vi "Winches Controller.vi"(8 "error in":errorcluster) -> ()   [LabVIEW 2019]
doc: "This VI executes continuously carrying out the current operation and responding to updates or new operations. It will often contain the timing or control code that is difficult to place directly in TeleOp. This VI generally opens all sensors and motors and isolates the rest of the robot code from knowing how the operations are carried out."
uses:
  <vilib>/Rock Robotics/WPI/Framework/Completion Status.ctl
  Winches Setpoints.ctl
  Winches Operations.ctl
  <vilib>/Rock Robotics/WPI/ThirdParty/Phoenix-LabVIEW/Motor Controller/Controls/CTRE_Phoenix_MotorControl_ControlMode.ctl
  Framework/Robot Global Data.vi
  <vilib>/Rock Robotics/Network Tables/NT Write Boolean.vi
panel:
  in  "Interactive Values":T1={"Operation"=enum."Actuate Lift", "Percent Power"=0.0}
  out "Current\nCmd":string
  in  "Buttons":cluster{"Execute Cmd":bool, "Abort Cmd":bool}
  out "Command Timing":cluster{"Start Time (ms)":u32, "Iterations":i32}
  out "Status":T3
  # "Tip: It may be helpful to observe inputs and sensor values.\nYou may also want to display tuning or debugging controls."
  # "Interactive Command: You may fill in the settings for a command\nand schedule it with the Execute button. You can observe and abort\nany command while fine tuning the code for the controller."
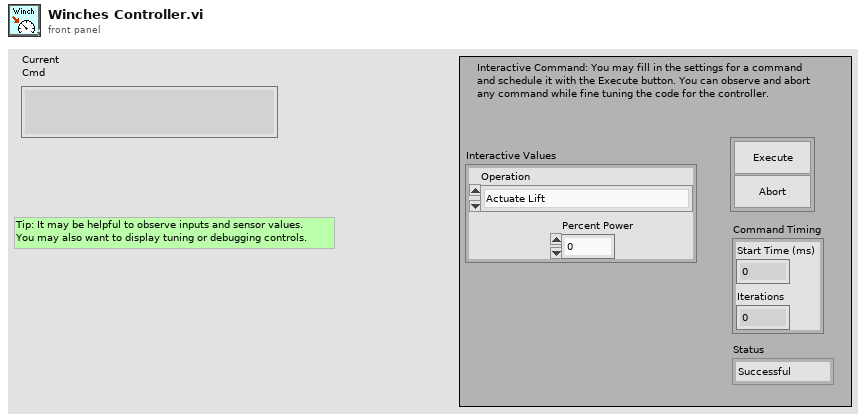
[diagram p1: front panel]
types:
  T1 = typedef "Winches Setpoints.ctl" = cluster{"Operation":T2, "Percent Power":dbl}
  T2 = typedef "Winches Operations.ctl" = enum16{"Reserve", "Read Current", "Actuate Lift", "Actuate Telescope"}
  T3 = typedef "Completion Status.ctl" = enum16{"Successful", "Aborted", "Incomplete"}
  T4 = typedef "WPI_MotorControlDeviceRef.ctl" = cluster{"DeviceStatus":errorcluster, "Type":T5, "PWM":cluster{"PWM Channel":T6, "DeadBand":T7}, "CAN":cluster{"Device Number":u8, "SetOutput VI Ref":variant, "GetOutput VI Ref":variant, "Enable VI Ref":variant, "Disable VI Ref":variant, "Data":variant}, "Invert":bool, "DIO PWM":cluster{"PWM \"Enable\" Channel":T6, "DIOChannel":T8, "PWM Rate":dbl}}
  T5 = typedef "WPI_MotorControlType.ctl" = enum16{"PWM", "CAN", "DIO PWM"}
  T6 = typedef "FPGA_DIOPWMChannel.ctl" = enum8{"PWM 0", "PWM 1", "PWM 2", "PWM 3", "PWM 4", "PWM 5", "PWM 6", "PWM 7", "PWM 8", "PWM 9", "PWM MXP 0", "PWM MXP 1", "PWM MXP 2", "PWM MXP 3", "PWM MXP 4", "PWM MXP 5", "PWM MXP 6", "PWM MXP 7", "PWM MXP 8", "PWM MXP 9", "Invalid"}
  T7 = typedef "WPI_PWMDeadband.ctl" = cluster{"Name":string, "maxPositivePwm":i32, "minPositivePwm":i32, "centerPwm":i32, "maxNegativePwm":i32, "minNegativePwm":i32, "angularRange":u16}
  T8 = typedef "FPGA_DIOChannel.ctl" = enum8{"DIO 0", "DIO 1", "DIO 2", "DIO 3", "DIO 4", "DIO 5", "DIO 6", "DIO 7", "DIO 8", "DIO 9", "DIO MXP 0", "DIO MXP 1", "DIO MXP 2", "DIO MXP 3", "DIO MXP 4", "DIO MXP 5", "DIO MXP 6", "DIO MXP 7", "DIO MXP 8", "DIO MXP 9", "DIO MXP 10", "DIO MXP 11", "DIO MXP 12", "DIO MXP 13", "DIO MXP 14", "DIO MXP 15", "SPI Port CS1", "SPI Port CS2", "SPI Port CS3", "SPI Port MISO", "SPI Port MOSI", "Invalid"}
  T9 = typedef "Command Status Info.ctl" = cluster{"Name":string, "Status":T3, "notifier out":T10}
  T10 = typedef "Completion Notifier.ctl" = refnum<notifier>
  T11 = cluster{"Current Command":T1, "Command Timing":cluster{"Start Time (ms)":u32, "Iterations":i32}, "Command Arguments":cluster{"Command Info":T9, "Description":string, "Default Command":T1, "queue out":refnum<queue>, "Subsystem Name":string}}
  T12 = typedef "CTRE_Phoenix_MotorControl_ControlMode.ctl" = u16
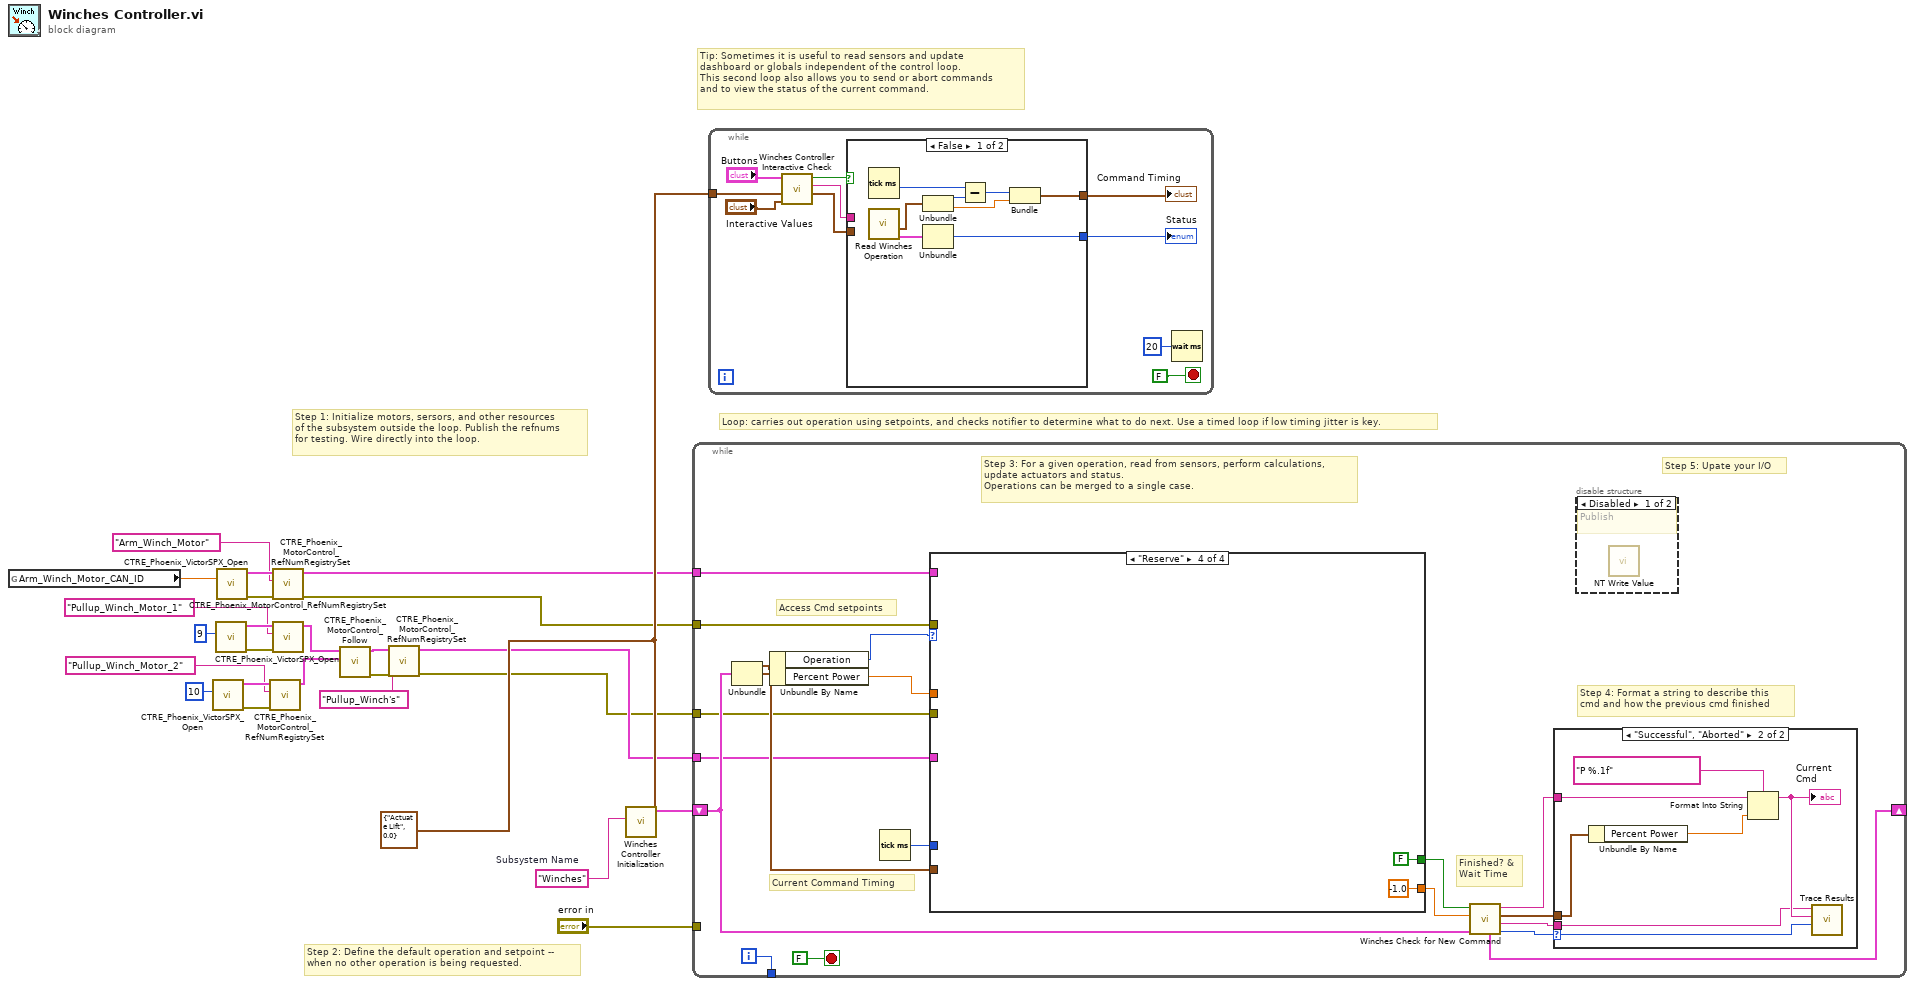
[diagram p0: block diagram]
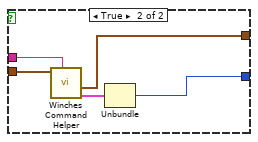
[diagram p2: hidden frame]
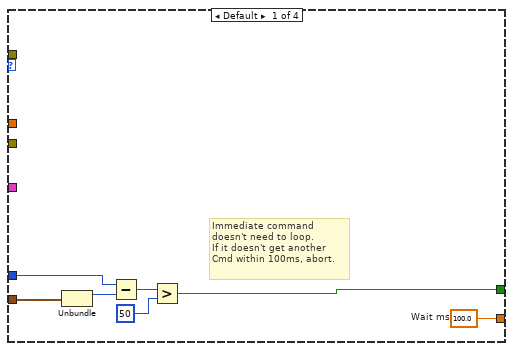
[diagram p5: hidden frame]
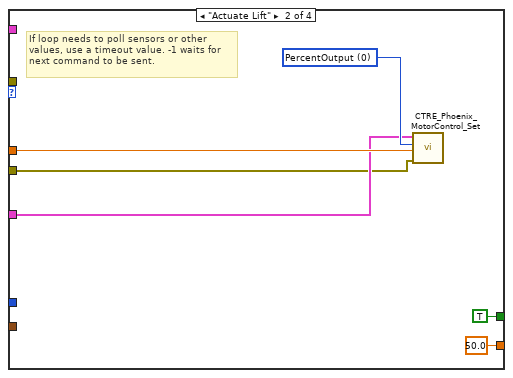
[diagram p6: hidden frame]
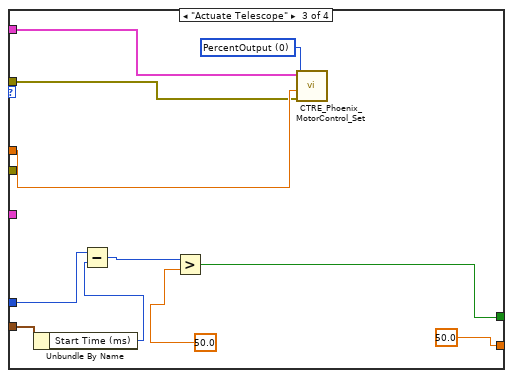
[diagram p7: hidden frame]
diagram:
  w12 = T1 {"Operation"=enum."Actuate Lift", "Percent Power"=0.0} ("Default Command")
  w23 = "Winches"  # Subsystem Name
  # "Tip: Sometimes it is useful to read sensors and update\ndashboard or globals independent of the control loop.\nThis second loop also allows you to send or abort commands\nand to view the status of the current command."
  # "Step 2: Define the default operation and setpoint --\nwhen no other operation is being requested."
  # "Step 1: Initialize motors, sersors, and other resources\nof the subsystem outside the loop. Publish the refnums\nfor testing. Wire directly into the loop."
  # "Loop: carries out operation using setpoints, and checks notifier to determine what to do next. Use a timed loop if low timing jitter is key."
  n1 = global read "Robot Global Data.vi" "Arm_Winch_Motor_CAN_ID"() -> (w22:dbl)
  n2 = call <vilib>:"CTRE_Phoenix_VictorSPX_Open.vi"("Device Number"=u8 10) -> ("error out"=w17:errorcluster, "CAN Talon SRX Ref"=w16:T4)  [unwired: 9 in]
  n3 = call <vilib>:"CTRE_Phoenix_VictorSPX_Open.vi"("Device Number"=u8 9) -> ("error out"=w19:errorcluster, "CAN Talon SRX Ref"=w18:T4)  [unwired: 9 in]
  n4 = call <vilib>:"CTRE_Phoenix_VictorSPX_Open.vi"("Device Number"=w22) -> ("error out"=w21:errorcluster, "CAN Talon SRX Ref"=w20:T4)  [unwired: 9 in]
  n5 = call <vilib>:"CTRE_Phoenix_MotorControl_RefNumRegistrySet.vi"("error in (no error)"=w17, "refnum name"="Pullup_Winch_Motor_2", "PhoenixMotorControlDevRef"=w16) -> ("PhoenixMotorControlDevRef"=w6:T4)  [unwired: 7 in, 1 out]
  n6 = call <vilib>:"CTRE_Phoenix_MotorControl_RefNumRegistrySet.vi"("error in (no error)"=w21, "refnum name"="Arm_Winch_Motor", "PhoenixMotorControlDevRef"=w20) -> ("error out"=w10:errorcluster, "PhoenixMotorControlDevRef"=w11:T4)  [unwired: 7 in]
  n7 = call <vilib>:"CTRE_Phoenix_MotorControl_RefNumRegistrySet.vi"("error in (no error)"=w19, "refnum name"="Pullup_Winch_Motor_1", "PhoenixMotorControlDevRef"=w18) -> ("PhoenixMotorControlDevRef"=w7:T4)  [unwired: 7 in, 1 out]
  n8 = call <vilib>:"CTRE_Phoenix_MotorControl_Follow.vi"("Master Controller to Follow"=w6, "PhoenixMotorControlDevRef"=w7) -> ("error out"=w5:errorcluster, "PhoenixMotorControlDevRef"=w4:T4)  [unwired: 8 in]
  n9 = call <vilib>:"CTRE_Phoenix_MotorControl_RefNumRegistrySet.vi"("error in (no error)"=w5, "refnum name"="Pullup_Winch's", "PhoenixMotorControlDevRef"=w4) -> ("error out"=w2:errorcluster, "PhoenixMotorControlDevRef"=w3:T4)  [unwired: 7 in]
  n10 = call "Winches Controller Initialization.vi"("Subsystem Name"=w23, "Default Command"=w12) -> ("Current Command"=w24:T11)  [unwired: 9 in]
  n11 = while {
    shift-right: [w40] -> _
    shift-left: w24 -> [w33]
    tunnel: [w43] -> _
    tunnel: "error in" -> [_]
    tunnel: w11 -> [w30]
    tunnel: w10 -> [w29]
    tunnel: w3 -> [w27]
    tunnel: w2 -> [w26]
    i -> [w43]
    stop <- FALSE stop-if-true
    # "Step 5: Upate your I/O"
    # "Step 4: Format a string to describe this\ncmd and how the previous cmd finished"
    # "Current Command Timing"
    # "Access Cmd setpoints"
    # "Finished? &\nWait Time"
    # "Step 3: For a given operation, read from sensors, perform calculations,\nupdate actuators and status.\nOperations can be merged to a single case."
    n12 = Unbundle(w33) -> ("Current Command"=w32:T1, "Command Timing"=w41:cluster{"Start Time (ms)":u32, "Iterations":i32})  [unwired: 1 out]
    n13 = Unbundle By Name(w32) -> ("Operation"=w31:T2, "Percent Power"=w28:dbl)
    n14 = Tick Count (ms)() -> (millisecond timer value=w42:u32)
    n15 = case shown="\"Reserve\"" w31 {
      tunnel: [w58 50.0 ("Wait ms") 50.0 -1.0 ("Wait ms")] -> w38
      tunnel: [w52 TRUE w71 FALSE] -> w39
      tunnel: w41 -> [w54 _ w69 _]
      tunnel: w42 -> [w53 _ w73 _]
      tunnel: w28 -> [_ w63 w75 _]
      tunnel: w30 -> [_ _ w66 _]
      tunnel: w29 -> [_ _ w65 _]
      tunnel: w27 -> [_ w60 _ _]
      tunnel: w26 -> [_ w59 _ _]
      frame Default {
        w58 = 100.0  # Wait ms
        # "Immediate command\ndoesn't need to loop.\nIf it doesn't get another\nCmd within 100ms, abort."
        n16 = Unbundle(w54) -> ("Start Time (ms)"=w57:u32)  [unwired: 1 out]
        n17 = Subtract(x=w53, y=w57) -> (x-y=w56:u32)
        n18 = Greater?(x=w56, y=u8 50 ("Left Motor")) -> (0:w52:bool)
      }
      frame "Actuate Lift" {
        w64 = T12 0 items=["PercentOutput"=0, "Position"=1, "Velocity"=2, "Current"=3, "Follower"=5, "MotionProfile"=6, "MotionMagic"=7, "MotionProfileArc"=10, "Disabled"=15] ("Control Mode")
        # "If loop needs to poll sensors or other\nvalues, use a timeout value. -1 waits for\nnext command to be sent."
        n19 = call <vilib>:"CTRE_Phoenix_MotorControl_Set.vi"("error in (no error)"=w59, "Output"=w63, "Control Mode"=w64, "PhoenixMotorControlDevRef"=w60) -> ()  [unwired: 6 in, 2 out]
      }
      frame "Actuate Telescope" {
        w74 = T12 0 items=["PercentOutput"=0, "Position"=1, "Velocity"=2, "Current"=3, "Follower"=5, "MotionProfile"=6, "MotionMagic"=7, "MotionProfileArc"=10, "Disabled"=15] ("Control Mode")
        n20 = Unbundle By Name(w69) -> ("Start Time (ms)"=w68:u32)
        n21 = Subtract(x=w73, y=w68) -> (x-y=w70:u32)
        n22 = Greater?(x=w70, y=50.0 ("x")) -> (0:w71:bool)
        n23 = call <vilib>:"CTRE_Phoenix_MotorControl_Set.vi"("error in (no error)"=w65, "Output"=w75, "Control Mode"=w74, "PhoenixMotorControlDevRef"=w66) -> ()  [unwired: 6 in, 2 out]
      }
      frame "Reserve" {
      }
    }
    n24 = call "Winches Check for New Command.vi"("Current Command"=w33, "Wait time (ms)"=w38, "Finished?"=w39) -> ("Completion"=w34:T3, "Subsystem Name"=w35:string, "Current Command"=w36:T1, "Initial Trace String"=w37:string, "NextCommand"=w40:T11)  [unwired: 4 in]
    n25 = case shown="\"Successful\", \"Aborted\"" w34 {
      selector: w34 -> [_ w51]
      tunnel: w37 -> [_ w48]
      tunnel: w36 -> [_ w49]
      tunnel: w35 -> [_ w46]
      frame "Incomplete", Default {
        # "Continuing current command"
      }
      frame "Successful", "Aborted" {
        # "Report and setup for next command"
        n26 = Unbundle By Name(w49) -> ("Percent Power"=w45:dbl)
        n27 = Format Into String(format string="P %.1f", initial string=w48, w45) -> (resulting string=w47:string)  [unwired: 1 in, 1 out]
        "Current\nCmd" <- w47
        n28 = call <vilib>:"Trace Results.vi"("Status of previous command"=w51, "Description"=w47, "Subsystem"=w46) -> ()  [unwired: 9 in]
      }
    }
    n29 = disable-structure shown="Disabled" {
      frame Disabled {
        # "Publish"
        n30 = call-poly <vilib>:"NT Write Value.vi"() -> ()  [unwired: 11 in, 1 out]
      }
      frame Enabled {
      }
    }
  }
  n31 = while {
    tunnel: w12 -> [w84]
    stop <- FALSE stop-if-true
    n32 = call "Winches Controller Interactive Check.vi"("Interactive Command in"="Interactive Values", "Default Command"=w84, "Buttons"="Buttons") -> ("Interactive Command out"=w81:T1, "Trace String"=w82:string, "Schedule"=w83:bool)  [unwired: 6 in]
    n33 = case shown="False" w83 {
      tunnel: [w95 w100] -> w80
      tunnel: w81 -> [_ w98]
      tunnel: [w91 w96] -> w79
      tunnel: w82 -> [_ w99]
      frame False {
        n34 = Tick Count (ms)() -> (millisecond timer value=w90:u32)
        n35 = call "Read Winches Operation.vi"() -> ("Command Info"=w88:T9, "SubSystem Data"=w89:T1)  [unwired: 9 in, 1 out]
        n36 = Unbundle(w89) -> ("Operation"=w94:T2, "Percent Power"=w92:dbl)
        n37 = Unbundle(w88) -> ("Status"=w95:T3)  [unwired: 2 out]
        n38 = Subtract(x=w90, y=w94) -> (x-y=w93:u32)
        n39 = Bundle(w93, "Percent Power"=w92) -> (w91:cluster{u32, "Percent Power":dbl})  [unwired: 1 in]
      }
      frame True {
        n40 = call "Winches Command Helper.vi"("Description"=w99, "SubSystem Data"=w98) -> ("Command Info Out"=w97:T9, "Command Timing"=w96:cluster{"Start Time (ms)":u32, "Iterations":i32})  [unwired: 7 in, 1 out]
        n41 = Unbundle(w97) -> ("Status"=w100:T3)  [unwired: 2 out]
      }
    }
    "Status" <- w80
    "Command Timing" <- w79
    n42 = Wait (ms)(milliseconds to wait=u32 20) -> ()  [unwired: 1 out]
  }
